vi "lvGetInstalledNISoftware.vi"   [LabVIEW 2014, in "lvcommonbuild.lvlib"]
uses:
  lvcommonbuild.lvlib
  <vilib>/nisyscfg/Component Types.ctl
  <vilib>/nisyscfg/Get Installed Components.vi
  <vilib>/nisyscfg/Close (System).vi
  <vilib>/nisyscfg/nisyscfg.lvlib
  <vilib>/Wiresmith Technology/LabVIEW CLI/CLI Class/CLI.lvclass
types:
  T1 = enum16{"open", "replace", "create", "open or create", "replace or create", "replace or create with confirmation"}
  T2 = typedef "nisyscfg.lvlib/Component Types.ctl" = u32
  T3 = typedef "nisyscfg.lvlib/Software 1.2.ctl" = cluster{"title":string, "description":string, "ID":string, "version":string, "component type":T4}
  T4 = typedef "nisyscfg.lvlib/Component Type.ctl" = u32
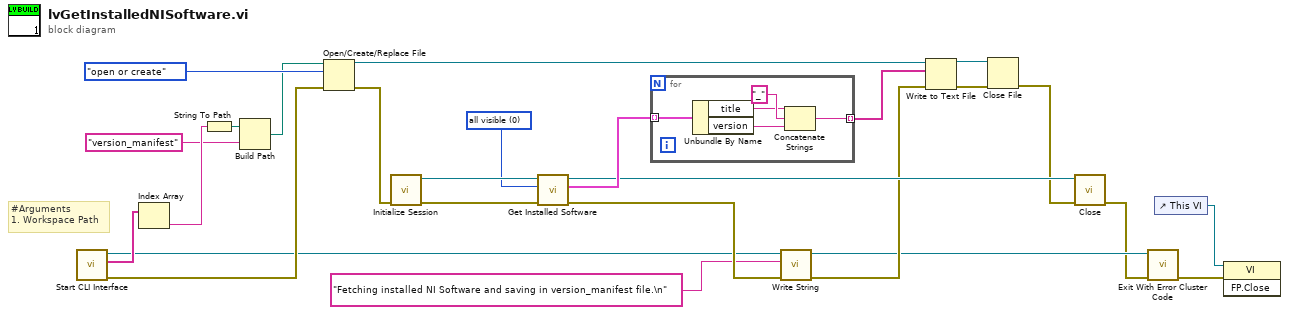
[diagram p0: block diagram]
diagram:
  w24 = T2 0 items=["all visible", "all including hidden", "standard only", "startup only"] ("Item Types (all visible)")
  # "#Arguments\n1. Workspace Path"
  n1 = call <vilib>:"Start CLI Interface.vi"() -> ("error out"=w9:errorcluster, "Custom Parameters"=w14:string[], "CLI out"=w6:refnum<class "CLI.lvclass">)  [unwired: 9 in]
  n2 = Index Array(array=w14) -> (element=w13:string)  [unwired: 1 in]
  n3 = String To Path(string=w13) -> (path=w12:path)
  n4 = Build Path(base path=w12, name or relative path="version_manifest") -> (appended path=w10:path)
  n5 = Open/Create/Replace File(file path (use dialog)=w10, error in=w9, operation (0:open)=T1."open or create") -> (refnum out=w18:refnum<file>, error out=w21:errorcluster)  [unwired: 3 in, 1 out]
  n6 = call <vilib>:"Initialize Session.vi"("error in (no error)"=w21) -> ("error out"=w26:errorcluster, "Session out"=w25:refnum<k21>)  [unwired: 9 in]
  n7 = call-poly <vilib>:"Get Installed Software.vi"("error in (no error)"=w26, "Item Types (all visible)"=w24, "Session in"=w25) -> ("error out"=w8:errorcluster, "Software Components"=w23:T3[], "Session out"=w22:refnum<k21>)  [unwired: 6 in]
  n8 = for {
    tunnel: w23 -> [w31] mode=indexing
    tunnel: [w27] -> w19 mode=indexing
    n9 = Unbundle By Name(w31) -> ("title"=w29:string, "version"=w28:string)
    n10 = Concatenate Strings(w29, "_" ("string"), w28) -> (w27:string)
  }
  n11 = call <vilib>:"Write String.vi"("error in (no error)"=w8, "Text to Write"="Fetching installed NI Software and saving in version_manifest file.\n", "CLI in"=w6) -> ("error out"=w7:errorcluster, "CLI out"=w4:refnum<class "CLI.lvclass">)  [unwired: 7 in]
  n12 = Write to Text File(file (use dialog)=w18, text=w19, error in=w7) -> (refnum out=w16:refnum<file>, error out=w17:errorcluster)  [unwired: 1 in, 1 out]
  n13 = Close File(refnum=w16, error in=w17) -> (error out=w15:errorcluster)  [unwired: 1 out]
  n14 = call-poly <vilib>:"Close.vi"("error in (no error)"=w15, "Session in"=w22) -> ("error out"=w3:errorcluster)  [unwired: 9 in]
  n15 = call <vilib>:"Exit With Error Cluster Code.vi"("error in (no error)"=w3, "CLI in"=w4) -> ("error out"=w2:errorcluster)  [unwired: 9 in]
  n16 = control-ref of="This VI"() -> (w1:refnum<vi>)
  n17 = invoke class="VI" method="FP.Close"(reference=w1, error in=w2) -> ()  [unwired: 1 in, 3 out]
